vi "Count.vi"(8 "error in (no error)":errorcluster caption="错误输入（无错误）", 11 "Queue 输入":refnum<class "Queue.lvclass"> caption="DNL_LabVIEW Object in") -> (0 "error out":errorcluster caption="错误输出", 3 "Queue 输出":refnum<class "Queue.lvclass"> caption="DNL_LabVIEW Object out")   [LabVIEW 2012, in "Queue.lvclass"]
uses:
  Queue.lvclass
  Queue.lvclass/Queue.ctl
panel:
  out "Count":i32
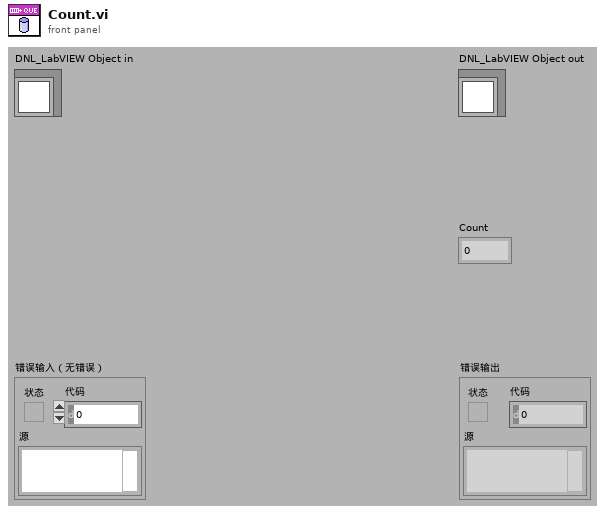
[diagram p1: front panel]
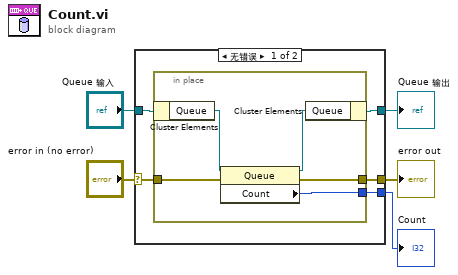
[diagram p0: block diagram]
diagram:
  n1 = case shown="无错误" "error in (no error)" {
    selector: "error in (no error)" -> [w7 w17]
    tunnel: [w6 w17] -> w4
    tunnel: [w8 w16] -> w2
    tunnel: "Queue 输入" -> [w10 w16]
    tunnel: [w9 _] -> w1
    frame No Error {
      n2 = in-place {
        in-place-border: [w13] -> w9
        in-place-border: w7 -> [w12]
        in-place-border: [w11] -> w6
        n3 = in-place-cluster #1(w10) -> ("Queue"=w15:refnum<k24>)
        n4 = property class="Queue"(reference=w15, error in=w12) -> (reference out=w14:refnum<k24>, error out=w11:errorcluster, "Count"=w13:i32)
        n5 = in-place-cluster #1("Queue"=w14) -> (w8:refnum<class "Queue.lvclass">)
      }
    }
    frame Error {
    }
  }
  "error out" <- w4
  "Queue 输出" <- w2
  "Count" <- w1
